vi "Free libssh2_knownhost.vi"(8 "error in (no error)":errorcluster, 11 "libssh2_knownhost*":u64) -> (0 "error out":errorcluster)   [LabVIEW 2013, in "libssh2.lvlib"]
uses:
  libssh2.lvlib
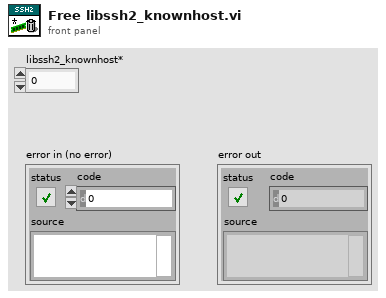
[diagram p1: front panel]
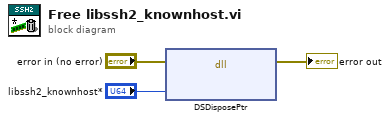
[diagram p0: block diagram]
diagram:
  n1 = dll-call lib="LabVIEW" fn="DSDisposePtr"(error in="error in (no error)", "p"="libssh2_knownhost*") -> (error out=→"error out":errorcluster)  [unwired: 4 in, 1 out]
